vi "平台接口对接.vi"() -> ()   [LabVIEW 2016]
uses:
  <vilib>/NI/Modbus Library/API/Wrapper/Create TCP Slave.vi
  <vilib>/NI/Modbus Library/API/slave/Modbus Slave.lvclass
  <vilib>/NI/Modbus Library/API/Wrapper/API Main.lvlib
panel:
  in  "运行间隔":i16=4 min=1 max=24
  in  "运行模式":enum16{"维护模式", "常规模式", "应急模式", "质控模式"}(ring)
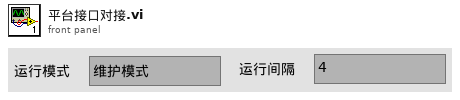
[diagram p1: front panel]
types:
  T1 = cluster{"启动参数":cluster{"氨氮":bool, "总磷":bool, "总氮":bool, "CODMn":bool, "CODCr":bool, "多参数":bool}, "运行模式":enum16{"维护模式", "常规模式", "应急模式", "质控模式"}, "质控频次":enum16{"关闭", "每天", "星期一", "星期二", "星期三", "星期四", "星期五", "星期六", "星期日"}, "空白核查时间":u16, "跨度核查时间":u16, "多参数测试间隔":u16, "湿化学测试间隔":u16}
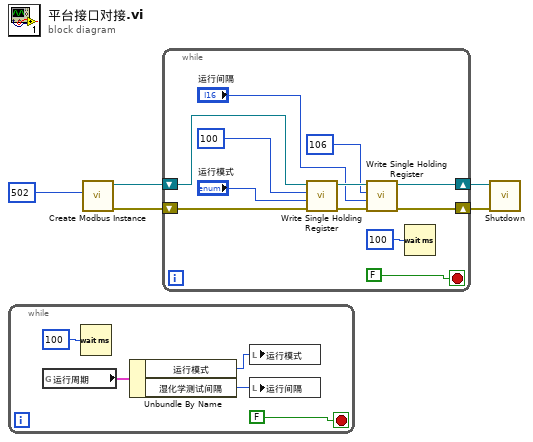
[diagram p0: block diagram]
diagram:
  n1 = while {
    stop <- FALSE stop-if-true
    n2 = global read "系统设置全局变量.vi" "运行周期"() -> (w7:T1)
    n3 = Wait (ms)(milliseconds to wait=u32 100 ("等待时间（毫秒）")) -> ()  [unwired: 1 out]
    n4 = Unbundle By Name(w7) -> ("运行模式"=w10:enum16{"维护模式", "常规模式", "应急模式", "质控模式"}, "湿化学测试间隔"=w6:u16)
    n5 = local write "运行模式"(w10) -> ()
    n6 = local write "运行间隔"(w6) -> ()
  }
  n7 = call-poly <vilib>:"Create Modbus Instance.vi"("port (502)"=u16 502) -> ("error out"=w3:errorcluster, "TCP slave instance"=w4:refnum<class "Modbus Slave.lvclass">)  [unwired: 9 in]
  n8 = while {
    shift-right: [w16] -> w2
    shift-left: w4 -> [w21]
    shift-right: [w17] -> w1
    shift-left: w3 -> [w20]
    stop <- FALSE stop-if-true
    n9 = call-dynamic "Write Single Holding Register.vi"("error in"=w20, "register to write"="运行模式", "address"=u16 100 ("starting address"), "Modbus slave in"=w21) -> ("error out"=w18:errorcluster, "Modbus slave out"=w19:refnum<class "Modbus Slave.lvclass">)  [unwired: 6 in]
    n10 = call-dynamic "Write Single Holding Register.vi"("error in"=w18, "register to write"="运行间隔", "address"=u16 106, "Modbus slave in"=w19) -> ("error out"=w17:errorcluster, "Modbus slave out"=w16:refnum<class "Modbus Slave.lvclass">)  [unwired: 6 in]
    n11 = Wait (ms)(milliseconds to wait=u32 100 ("等待时间（毫秒）")) -> ()  [unwired: 1 out]
  }
  n12 = call-dynamic "Shutdown.vi"("error in"=w1, "Modbus slave in"=w2) -> ()  [unwired: 9 in, 1 out]
